vi "ConfigureTalonsAuto.vi"(8 "Pigeon Talon":T1, 9 "Pigeon":T6 {"Type" items=["CAN"=352321536, "TalonSRX"=33554432]}, 10 "Right Side":T1, 11 "Left Side":T1) -> ()   [LabVIEW 2017]
uses:
  Constants.vi
  <vilib>/Rock Robotics/WPI/ThirdParty/Phoenix-LabVIEW/Motor Controller/Controls/CTRE_Phoenix_MotorControl_FeedbackDevice.ctl
  <vilib>/Rock Robotics/WPI/ThirdParty/Phoenix-LabVIEW/Motor Controller/Controls/CTRE_Phoenix_MotorControl_RemoteSourceType.ctl
  <vilib>/Rock Robotics/WPI/ThirdParty/Phoenix-LabVIEW/Motor Controller/Controls/CTRE_Phoenix_MotorControl_SensorTermFeedbackDevice_Enhanced.ctl
  <vilib>/Rock Robotics/WPI/ThirdParty/Phoenix-LabVIEW/Motor Controller/Controls/CTRE_Phoenix_MotorControl_StatusFrameEnhanced.ctl
  <vilib>/Rock Robotics/WPI/ThirdParty/Phoenix-LabVIEW/Motor Controller/Controls/CTRE_Phoenix_MotorControl_ControlMode.ctl
  <vilib>/Rock Robotics/WPI/ThirdParty/Phoenix-LabVIEW/Pigeon IMU/CTRE_PigeonIMU_ConnectionType.ctl
  <vilib>/Rock Robotics/WPI/ThirdParty/Phoenix-LabVIEW/Pigeon IMU/CTRE_PigeonIMU_DeviceRef.ctl
  <vilib>/Rock Robotics/SystemInterfaces/DIO/FPGA_DIOPWMChannel.ctl
  <vilib>/Rock Robotics/WPI/PWM/WPI_PWMDeadband.ctl
  <vilib>/Rock Robotics/WPI/MotorControl/WPI_MotorControlType.ctl
  <vilib>/Rock Robotics/SystemInterfaces/DIO/FPGA_DIOChannel.ctl
  <vilib>/Rock Robotics/WPI/MotorControl/WPI_MotorControlDeviceRef.ctl
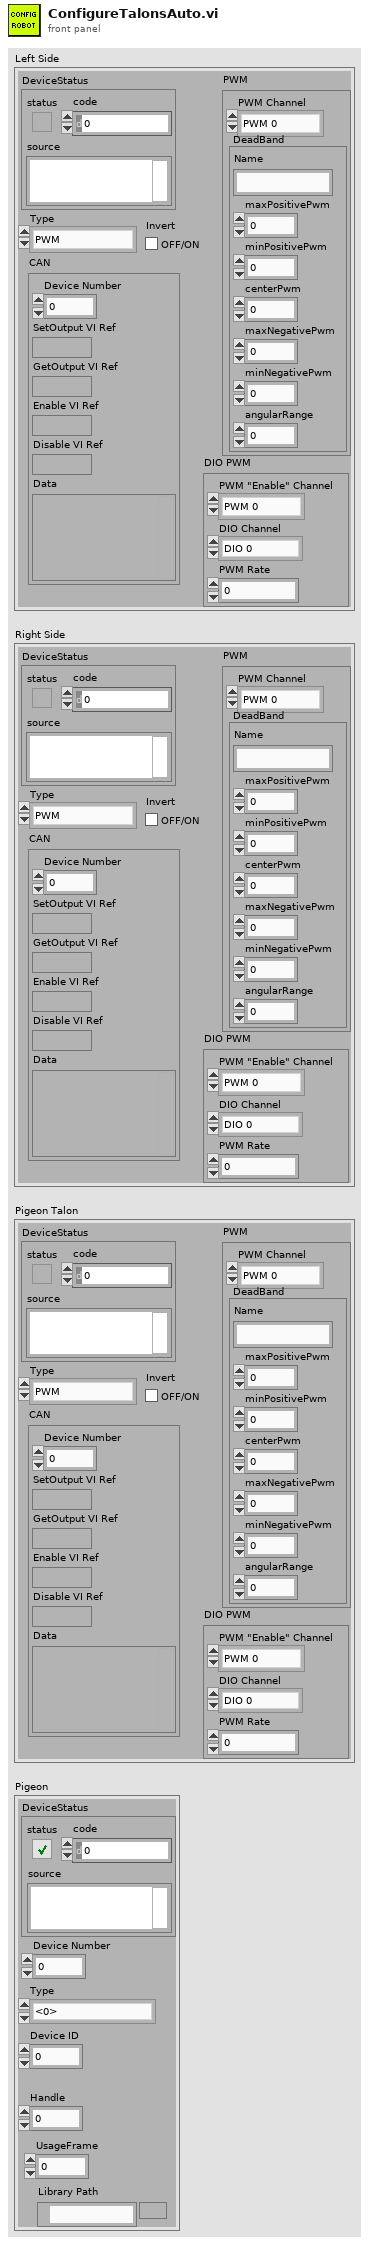
[diagram p1: front panel]
types:
  T1 = typedef "WPI_MotorControlDeviceRef.ctl" = cluster{"DeviceStatus":errorcluster, "Type":T2, "PWM":cluster{"PWM Channel":T3, "DeadBand":T4}, "CAN":cluster{"Device Number":u8, "SetOutput VI Ref":variant, "GetOutput VI Ref":variant, "Enable VI Ref":variant, "Disable VI Ref":variant, "Data":variant}, "Invert":bool, "DIO PWM":cluster{"PWM \"Enable\" Channel":T3, "DIOChannel":T5, "PWM Rate":dbl}}
  T2 = typedef "WPI_MotorControlType.ctl" = enum16{"PWM", "CAN", "DIO PWM"}
  T3 = typedef "FPGA_DIOPWMChannel.ctl" = enum8{"PWM 0", "PWM 1", "PWM 2", "PWM 3", "PWM 4", "PWM 5", "PWM 6", "PWM 7", "PWM 8", "PWM 9", "PWM MXP 0", "PWM MXP 1", "PWM MXP 2", "PWM MXP 3", "PWM MXP 4", "PWM MXP 5", "PWM MXP 6", "PWM MXP 7", "PWM MXP 8", "PWM MXP 9", "Invalid"}
  T4 = typedef "WPI_PWMDeadband.ctl" = cluster{"Name":string, "maxPositivePwm":i32, "minPositivePwm":i32, "centerPwm":i32, "maxNegativePwm":i32, "minNegativePwm":i32, "angularRange":u16}
  T5 = typedef "FPGA_DIOChannel.ctl" = enum8{"DIO 0", "DIO 1", "DIO 2", "DIO 3", "DIO 4", "DIO 5", "DIO 6", "DIO 7", "DIO 8", "DIO 9", "DIO MXP 0", "DIO MXP 1", "DIO MXP 2", "DIO MXP 3", "DIO MXP 4", "DIO MXP 5", "DIO MXP 6", "DIO MXP 7", "DIO MXP 8", "DIO MXP 9", "DIO MXP 10", "DIO MXP 11", "DIO MXP 12", "DIO MXP 13", "DIO MXP 14", "DIO MXP 15", "SPI Port CS1", "SPI Port CS2", "SPI Port CS3", "SPI Port MISO", "SPI Port MOSI", "Invalid"}
  T6 = typedef "CTRE_PigeonIMU_DeviceRef.ctl" = cluster{"DeviceStatus":errorcluster, "Device Number":u8, "Type":T7, "Device ID":u32, "Handle":u64, "UsageFrame":u32, "Library Path":path}
  T7 = typedef "CTRE_PigeonIMU_ConnectionType.ctl" = u32
  T8 = typedef "CTRE_Phoenix_MotorControl_ControlMode.ctl" = u16
  T9 = typedef "CTRE_Phoenix_MotorControl_StatusFrameEnhanced.ctl" = u16
  T10 = typedef "CTRE_Phoenix_MotorControl_FeedbackDevice.ctl" = i8
  T11 = typedef "CTRE_Phoenix_MotorControl_SensorTermFeedbackDevice_Enhanced.ctl" = i8
  T12 = typedef "CTRE_Phoenix_MotorControl_RemoteSourceType.ctl" = enum16{"Off", "Talon SRX Selected Sensor", "Pigeon IMU Yaw", "Pigeon IMU Pitch", "Pigeon IMU Roll", "CANifier Quadrature", "CANifier PWM Input 0", "CANifier PWM Input 1", "CANifier PWM Input 2", "CANifier PWM Input 3", "Gadgeteer Pigeon Yaw", "Gadgeteer Pigeon Pitch", "Gadgeteer Pigeon Roll"}
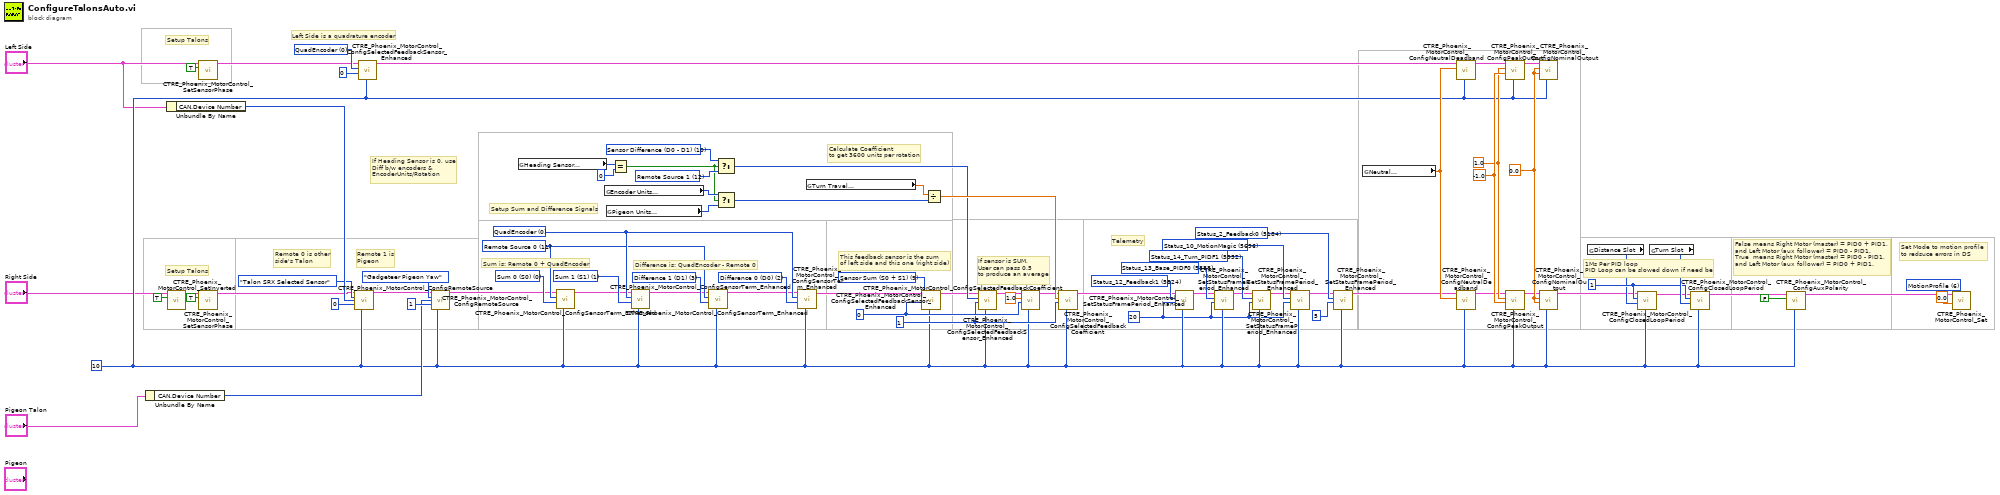
[diagram p0: block diagram]
diagram:
  w9 = 10
  w50 = 1
  w79 = 0
  w7 = T8 6 items=["PercentOutput"=0, "Position"=1, "Velocity"=2, "Current"=3, "Follower"=5, "MotionProfile"=6, "MotionMagic"=7, "MotionProfileArc"=10, "Disabled"=15] ("Control Mode")
  w77 = 1 ("loopTimeMs")
  w74 = 0.0 ("Forward Nominal Percent Output")
  w71 = -1.0 ("Reverse Peak Percent Output")
  w70 = 1.0 ("Forward Peak Percent Output")
  w3 = 20 ("periodMs")
  w63 = T9 5184 items=["Status_1_General"=5120, "Status_2_Feedback0"=5184, "Status_3_Quadrature"=5248, "Status_4_AinTempVbat"=5312, "Status_6_Misc"=5440, "Status_7_CommStatus"=5504, "Status_8_PulseWidth"=5568, "Status_9_MotProfBuffer"=5632, "Status_10_MotionMagic"=5696, "Status_11_UartGadgeteer"=5760, "Status_12_Feedback1"=5824, "Status_13_Base_PIDF0"=5888, "Status_14_Turn_PIDF1"=5952, "Status_15_FirmwareApiStatus"=6016] ("Status Frame")
  w62 = T9 5696 items=["Status_1_General"=5120, "Status_2_Feedback0"=5184, "Status_3_Quadrature"=5248, "Status_4_AinTempVbat"=5312, "Status_6_Misc"=5440, "Status_7_CommStatus"=5504, "Status_8_PulseWidth"=5568, "Status_9_MotProfBuffer"=5632, "Status_10_MotionMagic"=5696, "Status_11_UartGadgeteer"=5760, "Status_12_Feedback1"=5824, "Status_13_Base_PIDF0"=5888, "Status_14_Turn_PIDF1"=5952, "Status_15_FirmwareApiStatus"=6016] ("Status Frame")
  w61 = T9 5952 items=["Status_1_General"=5120, "Status_2_Feedback0"=5184, "Status_3_Quadrature"=5248, "Status_4_AinTempVbat"=5312, "Status_6_Misc"=5440, "Status_7_CommStatus"=5504, "Status_8_PulseWidth"=5568, "Status_9_MotProfBuffer"=5632, "Status_10_MotionMagic"=5696, "Status_11_UartGadgeteer"=5760, "Status_12_Feedback1"=5824, "Status_13_Base_PIDF0"=5888, "Status_14_Turn_PIDF1"=5952, "Status_15_FirmwareApiStatus"=6016] ("Status Frame")
  w60 = T9 5888 items=["Status_1_General"=5120, "Status_2_Feedback0"=5184, "Status_3_Quadrature"=5248, "Status_4_AinTempVbat"=5312, "Status_6_Misc"=5440, "Status_7_CommStatus"=5504, "Status_8_PulseWidth"=5568, "Status_9_MotProfBuffer"=5632, "Status_10_MotionMagic"=5696, "Status_11_UartGadgeteer"=5760, "Status_12_Feedback1"=5824, "Status_13_Base_PIDF0"=5888, "Status_14_Turn_PIDF1"=5952, "Status_15_FirmwareApiStatus"=6016] ("Status Frame")
  w59 = T9 5824 items=["Status_1_General"=5120, "Status_2_Feedback0"=5184, "Status_3_Quadrature"=5248, "Status_4_AinTempVbat"=5312, "Status_6_Misc"=5440, "Status_7_CommStatus"=5504, "Status_8_PulseWidth"=5568, "Status_9_MotProfBuffer"=5632, "Status_10_MotionMagic"=5696, "Status_11_UartGadgeteer"=5760, "Status_12_Feedback1"=5824, "Status_13_Base_PIDF0"=5888, "Status_14_Turn_PIDF1"=5952, "Status_15_FirmwareApiStatus"=6016] ("Status Frame")
  w44 = T10 12 items=["None"=-1, "QuadEncoder"=0, "Analog"=2, "Tachometer"=4, "Pulse Width Encoded Position"=8, "Sensor Sum (S0 + S1)"=9, "Sensor Difference (D0 - D1)"=10, "Remote Source 0"=11, "Remote Source 1"=12, "Software Emulated"=15] ("Feedback Device")
  w43 = T10 10 items=["None"=-1, "QuadEncoder"=0, "Analog"=2, "Tachometer"=4, "Pulse Width Encoded Position"=8, "Sensor Sum (S0 + S1)"=9, "Sensor Difference (D0 - D1)"=10, "Remote Source 0"=11, "Remote Source 1"=12, "Software Emulated"=15] ("Feedback Device")
  w37 = T10 9 items=["None"=-1, "QuadEncoder"=0, "Analog"=2, "Tachometer"=4, "Pulse Width Encoded Position"=8, "Sensor Sum (S0 + S1)"=9, "Sensor Difference (D0 - D1)"=10, "Remote Source 0"=11, "Remote Source 1"=12, "Software Emulated"=15] ("Feedback Device")
  w35 = u16 2 items=["Sum 0 (S0)", "Sum 1 (S1)", "Difference 0 (D0)", "Difference 1 (D1)"] ("Sensor Term")
  w34 = u16 3 items=["Sum 0 (S0)", "Sum 1 (S1)", "Difference 0 (D0)", "Difference 1 (D1)"] ("Sensor Term")
  w29 = u16 1 items=["Sum 0 (S0)", "Sum 1 (S1)", "Difference 0 (D0)", "Difference 1 (D1)"] ("Sensor Term")
  w33 = T11 0 items=["None"=-1, "QuadEncoder"=0, "Analog"=2, "Tachometer"=4, "Pulse Width Encoded Position"=8, "Remote Source 0"=11, "Remote Source 1"=12, "Software Emulated"=15] ("Feedback Device")
  w27 = u16 0 items=["Sum 0 (S0)", "Sum 1 (S1)", "Difference 0 (D0)", "Difference 1 (D1)"] ("Sensor Term")
  w32 = T11 11 items=["None"=-1, "QuadEncoder"=0, "Analog"=2, "Tachometer"=4, "Pulse Width Encoded Position"=8, "Remote Source 0"=11, "Remote Source 1"=12, "Software Emulated"=15] ("Feedback Device")
  w16 = T10 0 items=["None"=-1, "QuadEncoder"=0, "Analog"=2, "Tachometer"=4, "Pulse Width Encoded Position"=8, "Sensor Sum (S0 + S1)"=9, "Sensor Difference (D0 - D1)"=10, "Remote Source 0"=11, "Remote Source 1"=12, "Software Emulated"=15] ("Feedback Device")
  # "Set Mode to motion profile\nto redsuce errors in DS"
  # "False means Right Motor (master) = PID0 + PID1, \nand Left Motor (aux follower) = PID0 - PID1.\nTrue  means Right Motor (master) = PID0 - PID1, \nand Left Motor (aux follower) = PID0 + PID1."
  # "1Ms Per PID loop\nPID Loop can be slowed down if need be"
  # "Setup Talons"
  # "Telemetry"
  # "If sensor is SUM,\nUser can pass 0.5\nto produce an average"
  # "Calculate Coefficient\nto get 3600 units per rotation"
  # "If Heading Sensor is 0, use \nDiff b/w encoders &\nEncoderUnits/Rotation"
  # "This feedback sensor is the sum\nof left side and this one (right side)"
  # "Difference is: QuadEncoder - Remote 0"
  # "Sum is: Remote 0 + QuadEncoder"
  # "Setup Sum and Difference Signals"
  # "Remote 1 is\nPigeon"
  # "Remote 0 is other\nside's Talon"
  # "Left Side is a quadrature encoder"
  # "Setup Talons"
  n1 = Unbundle By Name("Pigeon Talon") -> ("CAN.Device Number"=w24:u8)
  n2 = Unbundle By Name("Left Side") -> ("CAN.Device Number"=w19:u8)
  n3 = call <vilib>:"CTRE_Phoenix_MotorControl_SetInverted.vi"("Invert?"=TRUE, "PhoenixMotorControlDevRef"="Right Side") -> ("PhoenixMotorControlDevRef"=w12:T1)  [unwired: 8 in, 1 out]
  n4 = call <vilib>:"CTRE_Phoenix_MotorControl_SetSensorPhase.vi"("PhaseSensor"=TRUE, "PhoenixMotorControlDevRef"="Left Side") -> ("PhoenixMotorControlDevRef"=w15:T1)  [unwired: 8 in, 1 out]
  n5 = call <vilib>:"CTRE_Phoenix_MotorControl_SetSensorPhase.vi"("PhaseSensor"=TRUE, "PhoenixMotorControlDevRef"=w12) -> ("PhoenixMotorControlDevRef"=w17:T1)  [unwired: 8 in, 1 out]
  n6 = call <vilib>:"CTRE_Phoenix_MotorControl_ConfigRemoteSource.vi"("PhoenixMotorControlDevRef"=w17, "Remote Device Type"=CTRE_Phoenix_MotorControl_RemoteSourceType."Talon SRX Selected Sensor", "Remote Device ID"=w19, "Source Index (0/1)"=0, "timeoutMs"=w9) -> ("PhoenixMotorControlDevRef"=w21:T1)  [unwired: 9 in, 1 out]
  n7 = call <vilib>:"CTRE_Phoenix_MotorControl_ConfigSelectedFeedbackSensor_Enhanced.vi"("timeoutMs"=w9, "pidLoopIdx"=0, "Feedback Device"=w16, "PhoenixMotorControlDevRef"=w15) -> ("PhoenixMotorControlDevRef"=w67:T1)  [unwired: 6 in, 1 out]
  n8 = call <vilib>:"CTRE_Phoenix_MotorControl_ConfigRemoteSource.vi"("PhoenixMotorControlDevRef"=w21, "Remote Device Type"=CTRE_Phoenix_MotorControl_RemoteSourceType."Gadgeteer Pigeon Yaw", "Remote Device ID"=w24, "Source Index (0/1)"=1, "timeoutMs"=w9) -> ("PhoenixMotorControlDevRef"=w26:T1)  [unwired: 9 in, 1 out]
  n9 = global read "Constants.vi" "Heading Sensor\nChoice"() -> (w38:i32)
  n10 = call <vilib>:"CTRE_Phoenix_MotorControl_ConfigSensorTerm_Enhanced.vi"("timeoutMs"=w9, "Sensor Term"=w27, "Feedback Device"=w32, "PhoenixMotorControlDevRef"=w26) -> ("PhoenixMotorControlDevRef"=w28:T1)  [unwired: 6 in, 1 out]
  n11 = global read "Constants.vi" "Encoder Units\nPer Rotation"() -> (w46:i32)
  n12 = global read "Constants.vi" "Pigeon Units\nPer Rotatoin"() -> (w45:i32)
  n13 = Equal?(x=w38, y=0) -> (x = y?=w40:bool)
  n14 = call <vilib>:"CTRE_Phoenix_MotorControl_ConfigSensorTerm_Enhanced.vi"("timeoutMs"=w9, "Sensor Term"=w29, "Feedback Device"=w33, "PhoenixMotorControlDevRef"=w28) -> ("PhoenixMotorControlDevRef"=w31:T1)  [unwired: 6 in, 1 out]
  n15 = call <vilib>:"CTRE_Phoenix_MotorControl_ConfigSensorTerm_Enhanced.vi"("timeoutMs"=w9, "Sensor Term"=w34, "Feedback Device"=w32, "PhoenixMotorControlDevRef"=w31) -> ("PhoenixMotorControlDevRef"=w30:T1)  [unwired: 6 in, 1 out]
  n16 = Select(t=w43, s=w40, f=w44) -> (s? t:f=w42:T10)
  n17 = Select(t=w46, s=w40, f=w45) -> (s? t:f=w51:i32)
  n18 = call <vilib>:"CTRE_Phoenix_MotorControl_ConfigSensorTerm_Enhanced.vi"("timeoutMs"=w9, "Sensor Term"=w35, "Feedback Device"=w33, "PhoenixMotorControlDevRef"=w30) -> ("PhoenixMotorControlDevRef"=w36:T1)  [unwired: 6 in, 1 out]
  n19 = global read "Constants.vi" "Turn Travel\nUnits Per Rotation"() -> (w52:dbl)
  n20 = call <vilib>:"CTRE_Phoenix_MotorControl_ConfigSelectedFeedbackSensor_Enhanced.vi"("timeoutMs"=w9, "pidLoopIdx"=w79, "Feedback Device"=w37, "PhoenixMotorControlDevRef"=w36) -> ("PhoenixMotorControlDevRef"=w41:T1)  [unwired: 6 in, 1 out]
  n21 = Divide(x=w52, y=w51) -> (x/y=w53:dbl)
  n22 = call <vilib>:"CTRE_Phoenix_MotorControl_ConfigSelectedFeedbackSensor_Enhanced.vi"("timeoutMs"=w9, "pidLoopIdx"=w50, "Feedback Device"=w42, "PhoenixMotorControlDevRef"=w41) -> ("PhoenixMotorControlDevRef"=w47:T1)  [unwired: 6 in, 1 out]
  n23 = call <vilib>:"CTRE_Phoenix_MotorControl_ConfigSelectedFeedbackCoefficient.vi"("timoutMs"=w9, "pidIdx"=w79, "coefficient"=1.0, "PhoenixMotorControlDevRef"=w47) -> ("PhoenixMotorControlDevRef"=w49:T1)  [unwired: 6 in, 1 out]
  n24 = call <vilib>:"CTRE_Phoenix_MotorControl_ConfigSelectedFeedbackCoefficient.vi"("timoutMs"=w9, "pidIdx"=w50, "coefficient"=w53, "PhoenixMotorControlDevRef"=w49) -> ("PhoenixMotorControlDevRef"=w54:T1)  [unwired: 6 in, 1 out]
  n25 = call <vilib>:"CTRE_Phoenix_MotorControl_SetStatusFramePeriod_Enhanced.vi"("timeoutMs"=w9, "periodMs"=w3, "Status Frame"=w59, "PhoenixMotorControlDevRef"=w54) -> ("PhoenixMotorControlDevRef"=w55:T1)  [unwired: 6 in, 1 out]
  n26 = call <vilib>:"CTRE_Phoenix_MotorControl_SetStatusFramePeriod_Enhanced.vi"("timeoutMs"=w9, "periodMs"=w3, "Status Frame"=w60, "PhoenixMotorControlDevRef"=w55) -> ("PhoenixMotorControlDevRef"=w56:T1)  [unwired: 6 in, 1 out]
  n27 = call <vilib>:"CTRE_Phoenix_MotorControl_SetStatusFramePeriod_Enhanced.vi"("timeoutMs"=w9, "periodMs"=w3, "Status Frame"=w61, "PhoenixMotorControlDevRef"=w56) -> ("PhoenixMotorControlDevRef"=w57:T1)  [unwired: 6 in, 1 out]
  n28 = call <vilib>:"CTRE_Phoenix_MotorControl_SetStatusFramePeriod_Enhanced.vi"("timeoutMs"=w9, "periodMs"=w3, "Status Frame"=w62, "PhoenixMotorControlDevRef"=w57) -> ("PhoenixMotorControlDevRef"=w58:T1)  [unwired: 6 in, 1 out]
  n29 = call <vilib>:"CTRE_Phoenix_MotorControl_SetStatusFramePeriod_Enhanced.vi"("timeoutMs"=w9, "periodMs"=5, "Status Frame"=w63, "PhoenixMotorControlDevRef"=w58) -> ("PhoenixMotorControlDevRef"=w65:T1)  [unwired: 6 in, 1 out]
  n30 = global read "Constants.vi" "Neutral\nDeadband"() -> (w68:dbl)
  n31 = call <vilib>:"CTRE_Phoenix_MotorControl_ConfigNeutralDeadband.vi"("timeoutMs"=w9, "Percent Deadband"=w68, "PhoenixMotorControlDevRef"=w67) -> ("PhoenixMotorControlDevRef"=w69:T1)  [unwired: 7 in, 1 out]
  n32 = call <vilib>:"CTRE_Phoenix_MotorControl_ConfigNeutralDeadband.vi"("timeoutMs"=w9, "Percent Deadband"=w68, "PhoenixMotorControlDevRef"=w65) -> ("PhoenixMotorControlDevRef"=w66:T1)  [unwired: 7 in, 1 out]
  n33 = call <vilib>:"CTRE_Phoenix_MotorControl_ConfigPeakOutput.vi"("timeoutMs"=w9, "Reverse Peak Percent Output"=w71, "Forward Peak Percent Output"=w70, "PhoenixMotorControlDevRef"=w69) -> ("PhoenixMotorControlDevRef"=w73:T1)  [unwired: 6 in, 1 out]
  n34 = call <vilib>:"CTRE_Phoenix_MotorControl_ConfigPeakOutput.vi"("timeoutMs"=w9, "Reverse Peak Percent Output"=w71, "Forward Peak Percent Output"=w70, "PhoenixMotorControlDevRef"=w66) -> ("PhoenixMotorControlDevRef"=w72:T1)  [unwired: 6 in, 1 out]
  n35 = call <vilib>:"CTRE_Phoenix_MotorControl_ConfigNominalOutput.vi"("timeoutMs"=w9, "Reverse Nominal Percent Output"=w74, "Forward Nominal Percent Output"=w74, "PhoenixMotorControlDevRef"=w73) -> ()  [unwired: 6 in, 2 out]
  n36 = call <vilib>:"CTRE_Phoenix_MotorControl_ConfigNominalOutput.vi"("timeoutMs"=w9, "Reverse Nominal Percent Output"=w74, "Forward Nominal Percent Output"=w74, "PhoenixMotorControlDevRef"=w72) -> ("PhoenixMotorControlDevRef"=w2:T1)  [unwired: 6 in, 1 out]
  n37 = global read "Constants.vi" "Distance Slot"() -> (w75:i32)
  n38 = call <vilib>:"CTRE_Phoenix_MotorControl_ConfigClosedLoopPeriod.vi"("timoutMs"=w9, "slotIdx"=w75, "loopTimeMs"=w77, "PhoenixMotorControlDevRef"=w2) -> ("PhoenixMotorControlDevRef"=w76:T1)  [unwired: 6 in, 1 out]
  n39 = global read "Constants.vi" "Turn Slot"() -> (w78:i32)
  n40 = call <vilib>:"CTRE_Phoenix_MotorControl_ConfigClosedLoopPeriod.vi"("timoutMs"=w9, "slotIdx"=w78, "loopTimeMs"=w77, "PhoenixMotorControlDevRef"=w76) -> ("PhoenixMotorControlDevRef"=w10:T1)  [unwired: 6 in, 1 out]
  n41 = call <vilib>:"CTRE_Phoenix_MotorControl_ConfigAuxPolarity.vi"("timeoutMs"=w9, "Invert"=FALSE, "PhoenixMotorControlDevRef"=w10) -> ("PhoenixMotorControlDevRef"=w5:T1)  [unwired: 8 in]
  n42 = call <vilib>:"CTRE_Phoenix_MotorControl_Set.vi"("Output"=0.0, "Control Mode"=w7, "PhoenixMotorControlDevRef"=w5) -> ()  [unwired: 7 in, 2 out]
